vi "RT Driver VI.vi"(7 "Operation":T1, 11 "Device Reference in":T2 format="%.0x") -> (0 "Error Code":i32)   [LabVIEW 2017, in "Waveform-Processing-Custom-Device Engine.lvlib"]
uses:
  Waveform-Processing-Custom-Device Engine.lvlib
  <vilib>/NI Veristand/Custom Device API/Custom Device Item Ref.ctl
  <vilib>/NI Veristand/Custom Device API/Hardware Interface Driver VI Operation.ctl
  RTStateVariables.ctl
  <vilib>/NI/NIVS Inline Async API/_VS Inline Async API/VS Inline Async API/VS Inline Async API.lvclass
  Shared/CompiledSettings.ctl
  <vilib>/NI Veristand/Custom Device API/Block Data Reference.ctl
  <vilib>/NI Veristand/Custom Device API/Data Reference.ctl
  <vilib>/NI Veristand/Custom Device API/Waveform Data Reference.ctl
  <vilib>/NI/NIVS Inline Async API/_VS Inline Async API/VS Inline Async API/VS Inline Async API.lvclass/VS Inline Async API.ctl
  <vilib>/NI/NIVS Inline Async API/_Data Access Engine/Data Access Engine/Data Access Engine.lvclass/Data Access Engine.ctl
  <vilib>/NI/NIVS Inline Async API/_Data Access Engine/Access Type Classes/Write/Write.lvclass/Write.ctl
  <vilib>/NI/NIVS Inline Async API/_Data Access Engine/Access Type Classes/ReadWrite/ReadWrite.lvclass/ReadWrite.ctl
  <vilib>/NI/NIVS Inline Async API/_Data Access Engine/Access Type Classes/Read/Read.lvclass/Read.ctl
  <vilib>/NI/NIVS Inline Async API/_Data Access Engine/Data Access Engine/Methods/Data.Engine.Read Data from HW.vi
  <vilib>/NI/NIVS Inline Async API/_VS Inline Async API/Error Handling Process/SubVIs/Error.GetError.vi
  <vilib>/NI/NIVS Inline Async API/_Data Access Engine/Data Access Engine/Methods/Data.Engine.Write Data to HW.vi
  <vilib>/NI/NIVS Inline Async API/_Data Access Engine/Access Type Classes/ReadWrite/ReadWrite.EngineData.vi
  <vilib>/NI/NIVS Inline Async API/_Data Access Engine/Access Type Classes/Write/Write.EngineData.vi
  <vilib>/NI/NIVS Inline Async API/_Data Access Engine/Access Type Classes/Read/Read.EngineData.vi
  <vilib>/NI Veristand/Custom Device API/NI VeriStand - Get Channel Value by Data Reference.vi
  <vilib>/NI Veristand/Custom Device API/NI VeriStand - Set Channel Value by Data Reference.vi
  <vilib>/NI Veristand/Custom Device API/NI VeriStand - Get Channel Values by Block Data Reference.vi
  Shared/Constants.vi
  <vilib>/NI Veristand/Custom Device API/Get Item Property (Variant).vi
  <vilib>/NI Veristand/Custom Device API/Global Data Refs.vi
  <vilib>/NI Veristand/Custom Device API/Custom Device API.lvlib
  <vilib>/NI VeriStand/Custom Device Tools/Custom Device Utility Library/Custom Device Utility Library.lvlib
  Shared/Waveform-Processing-Custom-Device Shared.lvlib
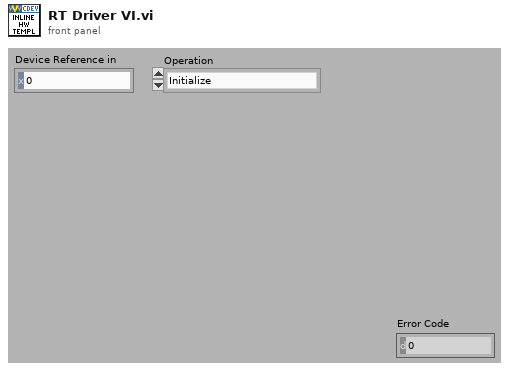
[diagram p1: front panel]
types:
  T1 = typedef "Custom Device API.lvlib/Hardware Interface Driver VI Operation.ctl" = enum16{"Initialize", "Start", "Read Data from HW", "Write Data to HW", "Close"}
  T2 = typedef "Custom Device API.lvlib/Custom Device Item Ref.ctl" = u64
  T3 = typedef "Waveform-Processing-Custom-Device Engine.lvlib/RTStateVariables.ctl" = cluster{"Async":refnum<class "VS Inline Async API.lvclass">, "Settings":T4}
  T4 = typedef "Waveform-Processing-Custom-Device Shared.lvlib/CompiledSettings.ctl" = cluster{"Name":string, "Buffer Length (samples)":u32, "Enable Array":bool[], "Parameter Block Data Refs":T5[], "Source Wfm Data Refs":T7[], "Result Wfm Data Refs":T7[], "Result Ch Data Refs":T6[], "Task Rate (Hz)":dbl}
  T5 = typedef "Custom Device API.lvlib/Block Data Reference.ctl" = cluster{"Data Reference":T6, "Offset":u64, "Length":u64}
  T6 = typedef "Custom Device API.lvlib/Data Reference.ctl" = i32
  T7 = typedef "Custom Device API.lvlib/Waveform Data Reference.ctl" = i32
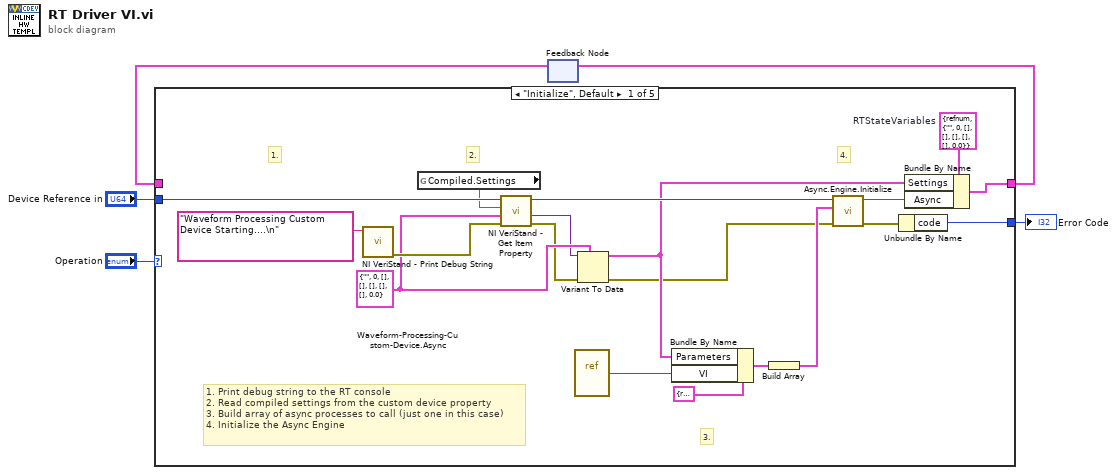
[diagram p0: block diagram]
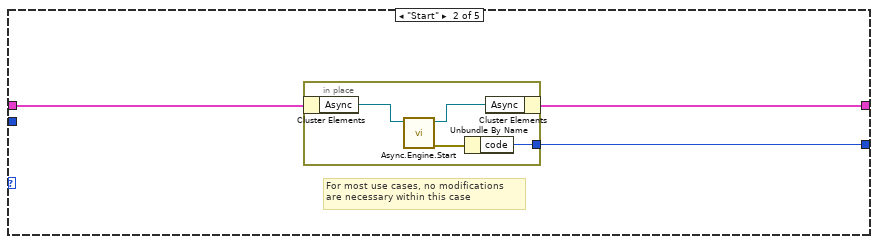
[diagram p2: hidden frame]
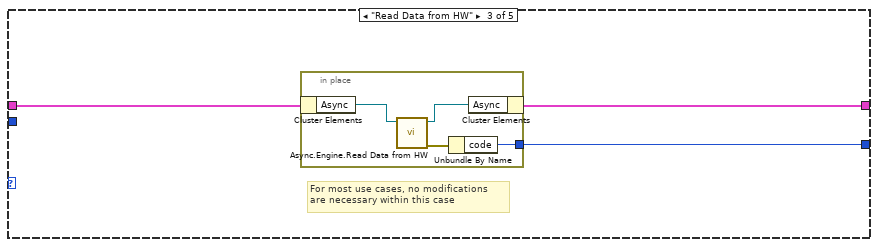
[diagram p3: hidden frame]
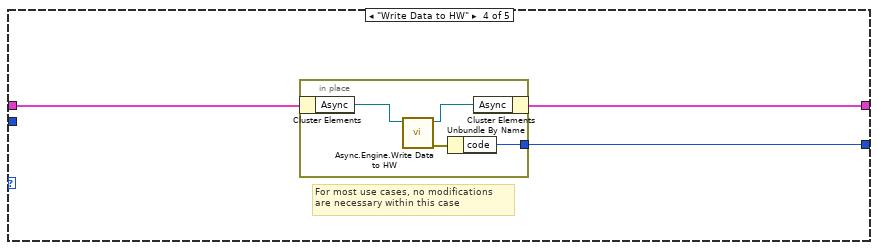
[diagram p4: hidden frame]
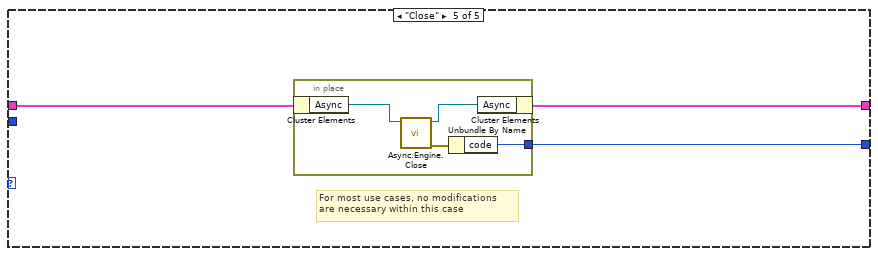
[diagram p5: hidden frame]
diagram:
  n1 = feedback #1() -> (w3:T3)  [unwired: 1 out]
  n2 = case shown="\"Initialize\", Default" "Operation" {
    tunnel: [w23 w26 w32 w39 w47] -> w4
    tunnel: w3 -> [_ w27 w34 w40 w48]
    tunnel: "Device Reference in" -> [w20 _ _ _ _]
    tunnel: [w12 w25 w33 w41 w46] -> w1
    frame "Initialize", Default {
      w13 = T4 {"Name"="", "Buffer Length (samples)"=0, "Enable Array"=[], "Parameter Block Data Refs"=[], "Source Wfm Data Refs"=[], "Result Wfm Data Refs"=[], "Result Ch Data Refs"=[], "Task Rate (Hz)"=0.0} ("CompiledSettings")
      w19 = T3 {"Async"=refnum, "Settings"={"Name"="", "Buffer Length (samples)"=0, "Enable Array"=[], "Parameter Block Data Refs"=[], "Source Wfm Data Refs"=[], "Result Wfm Data Refs"=[], "Result Ch Data Refs"=[], "Task Rate (Hz)"=0.0}}  # RTStateVariables
      # "2."
      # "3."
      # "4."
      # "1."
      # "1. Print debug string to the RT console\n2. Read compiled settings from the custom device property\n3. Build array of async processes to call (just one in this case)\n4. Initialize the Async Engine"
      n3 = call <vilib>:"NI VeriStand - Print Debug String.vi"("Message"="Waveform Processing Custom Device Starting....\n") -> ("error out"=w16:errorcluster)  [unwired: 10 in]
      n4 = global read "Constants.vi" "Compiled.Settings"() -> (w9:string)
      n5 = call-poly <vilib>:"NI VeriStand - Get Item Property.vi"("error in (no error)"=w16, "Default Value"=w13, "Property Name"=w9, "Item Ref in"=w20) -> ("error out"=w11:errorcluster, "Value"=w10:variant, "Item Ref out"=w17:T2)  [unwired: 4 in, 1 out]
      n6 = vi-ref "Waveform-Processing-Custom-Device.Async.vi"() -> (w14:refnum<vi>)
      n7 = Variant To Data(error in=w11, type=w13, Variant=w10) -> (data=w8:T4, error out=w7:errorcluster)
      n8 = Bundle By Name(cluster=cluster{"VI":refnum<vi>, "Parameters":variant} {"VI"=refnum, "Parameters"=variant} ("Process"), "Parameters"=w8, "VI"=w14) -> (w21:cluster{"VI":refnum<vi>, "Parameters":variant})
      n9 = Build Array(w21) -> (w18:cluster{"VI":refnum<vi>, "Parameters":variant}[])
      n10 = call <vilib>:"Async.Engine.Initialize.vi"("error in (no error)"=w7, "Processes"=w18, "Custom Device Ref"=w17) -> ("error out"=w6:errorcluster, "Async"=w24:refnum<class "VS Inline Async API.lvclass">)  [unwired: 7 in]
      n11 = Unbundle By Name(w6) -> ("code"=w12:i32)
      n12 = Bundle By Name(cluster=w19, "Settings"=w8, "Async"=w24) -> (w23:T3)
    }
    frame "Start" {
      # "For most use cases, no modifications \nare necessary within this case"
      n13 = in-place {
        in-place-border: [w28] -> w25
        n14 = in-place-cluster #2(w27) -> ("Async"=w31:refnum<class "VS Inline Async API.lvclass">)
        n15 = call <vilib>:"Async.Engine.Start.vi"("VS Inline Async API in"=w31) -> ("error out"=w29:errorcluster, "VS Inline Async API out"=w30:refnum<class "VS Inline Async API.lvclass">)  [unwired: 9 in]
        n16 = Unbundle By Name(w29) -> ("code"=w28:i32)
        n17 = in-place-cluster #2("Async"=w30) -> (w26:T3)
      }
    }
    frame "Read Data from HW" {
      # "For most use cases, no modifications \nare necessary within this case"
      n18 = in-place {
        in-place-border: [w36] -> w33
        n19 = in-place-cluster #3(w34) -> ("Async"=w38:refnum<class "VS Inline Async API.lvclass">)
        n20 = call <vilib>:"Async.Engine.Read Data from HW.vi"("Async in"=w38) -> ("error out"=w35:errorcluster, "Async out"=w37:refnum<class "VS Inline Async API.lvclass">)  [unwired: 9 in]
        n21 = Unbundle By Name(w35) -> ("code"=w36:i32)
        n22 = in-place-cluster #3("Async"=w37) -> (w32:T3)
      }
    }
    frame "Write Data to HW" {
      # "For most use cases, no modifications \nare necessary within this case"
      n23 = in-place {
        in-place-border: [w45] -> w41
        n24 = in-place-cluster #4(w40) -> ("Async"=w43:refnum<class "VS Inline Async API.lvclass">)
        n25 = call <vilib>:"Async.Engine.Write Data to HW.vi"("VS Inline Async API in"=w43) -> ("error out"=w44:errorcluster, "VS Inline Async API out"=w42:refnum<class "VS Inline Async API.lvclass">)  [unwired: 9 in]
        n26 = Unbundle By Name(w44) -> ("code"=w45:i32)
        n27 = in-place-cluster #4("Async"=w42) -> (w39:T3)
      }
    }
    frame "Close" {
      # "For most use cases, no modifications \nare necessary within this case"
      n28 = in-place {
        in-place-border: [w50] -> w46
        n29 = in-place-cluster #5(w48) -> ("Async"=w52:refnum<class "VS Inline Async API.lvclass">)
        n30 = call <vilib>:"Async.Engine.Close.vi"("Async in"=w52) -> ("error out"=w49:errorcluster, "Async out"=w51:refnum<class "VS Inline Async API.lvclass">)  [unwired: 9 in]
        n31 = Unbundle By Name(w49) -> ("code"=w50:i32)
        n32 = in-place-cluster #5("Async"=w51) -> (w47:T3)
      }
    }
  }
  "Error Code" <- w1
  n33 = feedback-in #1(w4) -> ()
